vi "Sort Channels by User.vi"(7 "Hardware Configuration":T1, 8 "error in":errorcluster, 10 "Waveforms in Read Order":waveform(dbl)[](array[waveform])) -> (0 "error out":errorcluster, 2 "Waveforms in User Order":waveform(dbl)[](array[waveform]))   [LabVIEW 2021, in "Load Frame.lvlib"]
uses:
  Load Frame.lvlib
  Acquisition/Acquisition.lvlib
  Acquisition/IO Device.ctl
  Acquisition/Sensor Type.ctl
  Acquisition/Channel Settings.ctl
  Interval Timer/Interval Length.ctl
  Interval Timer/Interval Timer.lvlib
  Interval Timer/Repeat Interval.ctl
  Interval Timer/Interval Token.ctl
  Acquisition/IO API.ctl
  Acquisition/IO Context.ctl
  Acquisition/Hardware Configuration.ctl
panel:
  out "found at":i32[](array[numeric])
  out "searching":string[](array[string])
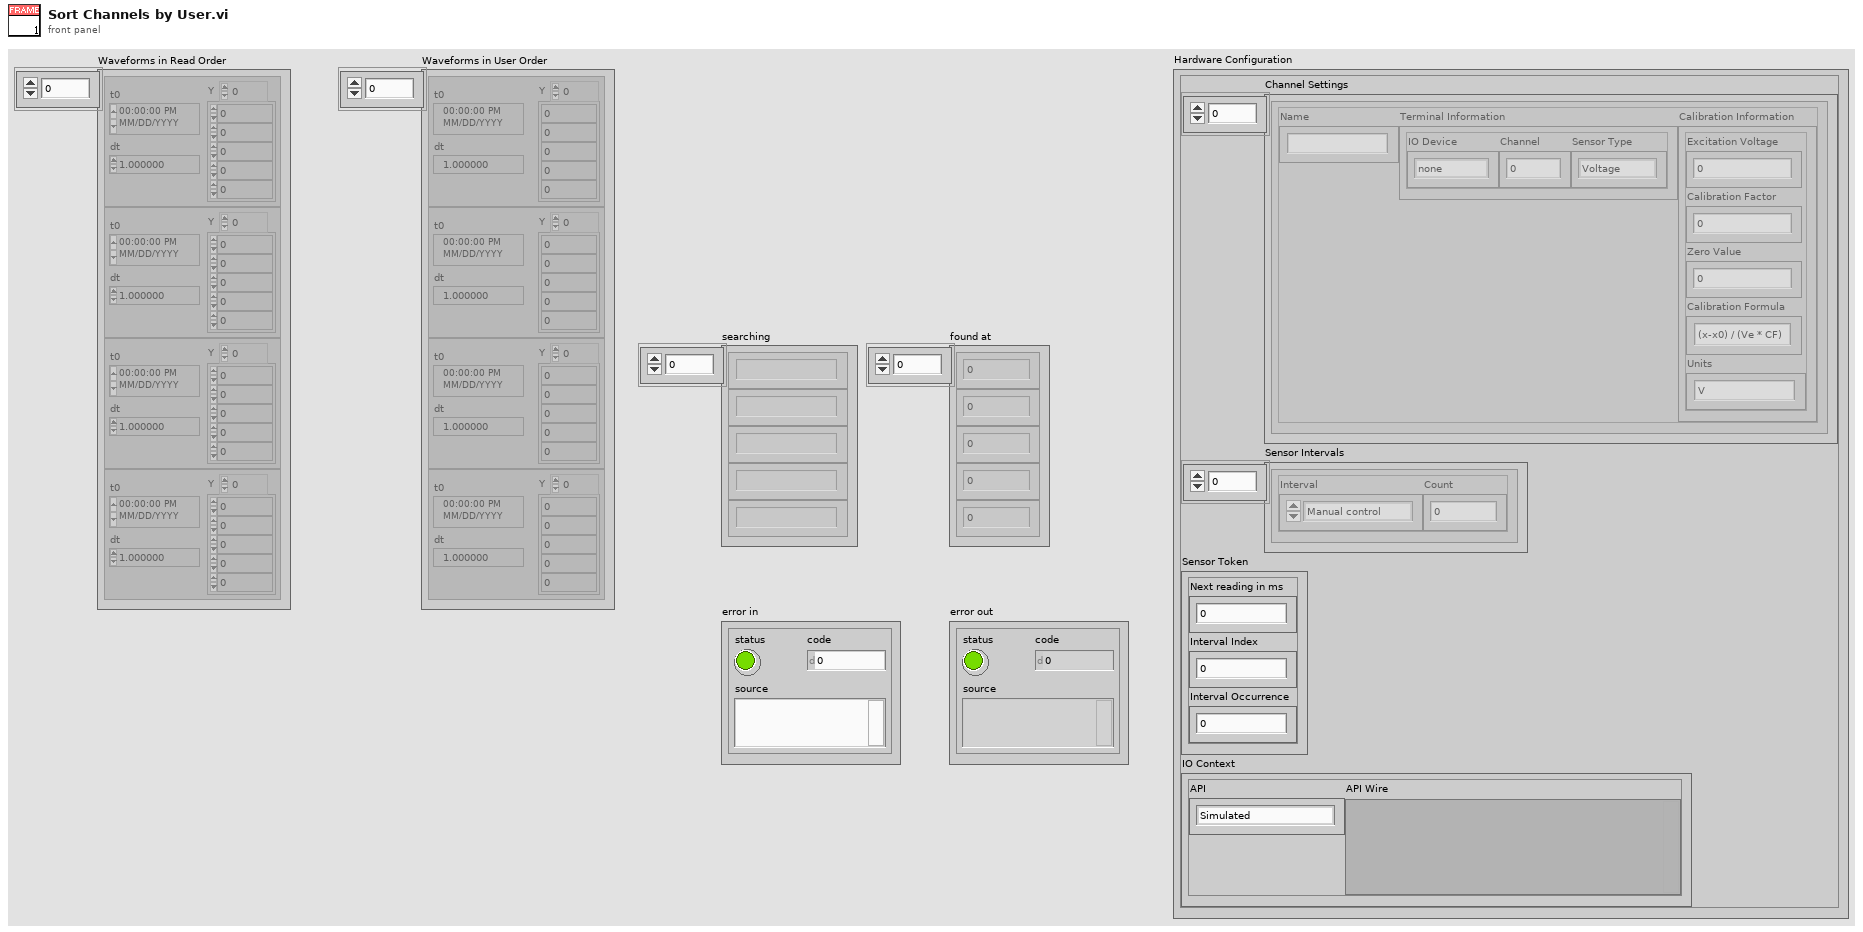
[diagram p1: front panel]
types:
  T1 = typedef "Acquisition.lvlib/Hardware Configuration.ctl" = cluster{"Channel Settings":T2[], "Sensor Intervals":T5[], "Sensor Token":T7, "IO Context":T8}
  T2 = typedef "Acquisition.lvlib/Channel Settings.ctl" = cluster{"Name":string, "Terminal Information":cluster{"IO Device":T3, "Channel":i32, "Sensor Type":T4}, "Calibration Information":cluster{"Excitation Voltage":dbl, "Calibration Factor":dbl, "Zero Value":dbl, "Calibration Formula":string, "Units":string}}
  T3 = typedef "Acquisition.lvlib/IO Device.ctl" = enum16{"none", "9219", "9401"}
  T4 = typedef "Acquisition.lvlib/Sensor Type.ctl" = enum16{"Voltage", "Load", "Pressure", "Encoder"}
  T5 = typedef "Interval Timer.lvlib/Repeat Interval.ctl" = cluster{"Interval":T6, "Count":i32}
  T6 = typedef "Interval Timer.lvlib/Interval Length.ctl" = enum16{"Manual control", "1 second", "10 seconds", "30 seconds", "60 seconds", "600 seconds", "1200 seconds", "3600 seconds"}
  T7 = typedef "Interval Timer.lvlib/Interval Token.ctl" = cluster{"Next reading in ms":u32, "Interval Index":i32, "Interval Occurrence":i32}
  T8 = typedef "Acquisition.lvlib/IO Context.ctl" = cluster{"API":T9, "API Wire":variant}
  T9 = typedef "Acquisition.lvlib/IO API.ctl" = enum16{"Simulated", "DAQmx"}
  T10 = typedef "Acquisition.lvlib/Acquired Data.ctl" = cluster{"Waveform Array":waveform(dbl)[]}
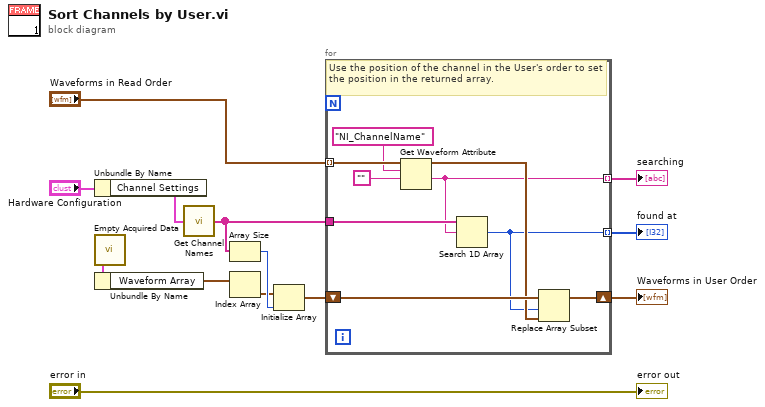
[diagram p0: block diagram]
diagram:
  n1 = Unbundle By Name("Hardware Configuration") -> ("Channel Settings"=w2:T2[])
  n2 = call "Empty Acquired Data.vi"() -> ("Empty Acquired Data"=w12:T10)
  n3 = Unbundle By Name(w12) -> ("Waveform Array"=w10:waveform(dbl)[])
  n4 = call "Get Channel Names.vi"("Channel Settings"=w2) -> ("Channel Names"=w1:string[])
  n5 = Array Size(array=w1) -> (size(s)=w13:i32)
  n6 = Index Array(array=w10) -> (element=w11:waveform(dbl))  [unwired: 1 in]
  n7 = Initialize Array(w11, w13) -> (w9:waveform(dbl)[])
  n8 = for {
    tunnel: "Waveforms in Read Order" -> [w22] mode=indexing
    tunnel: w1 -> [w19]
    tunnel: [w15] -> w8 mode=indexing
    tunnel: [w14] -> w7 mode=indexing
    shift-right: [w17] -> w6
    shift-left: w9 -> [w18]
    # "Use the position of the channel in the User's order to set the position in the returned array."
    n9 = Get Waveform Attribute(5:"", 6:"NI_ChannelName" ("name"), 7:w22) -> (1:w15:string, 3:w16:waveform(dbl))  [unwired: 1 in, 2 out]
    n10 = Search 1D Array(1D array=w19, element=w15) -> (index of element=w14:i32)  [unwired: 1 in]
    n11 = Replace Array Subset(array=w18, new element=w16, index=w14) -> (w17:waveform(dbl)[])
  }
  "searching" <- w8
  "found at" <- w7
  "Waveforms in User Order" <- w6
  "error out" <- "error in"
